vi "Create Space Image.vi"() -> ()   [LabVIEW 2020, in "Reversi.lvlib" / "Reversi.lvclass"]
uses:
  Reversi.lvclass
  Reversi.lvclass/Reversi.ctl
panel:
  out "White Space":picture
  out "Black Space":picture
  out "Blank Space":picture
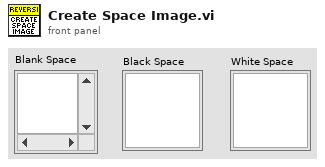
[diagram p1: front panel]
types:
  T1 = cluster{"left":i16, "top":i16, "right":i16, "bottom":i16}
  T2 = typedef "imagedata.ctl" = cluster{"image type":i32, "image depth":i32, "image":u8[], "mask":u8[], "colors":u32[], "Rectangle":cluster{"left":i16, "top":i16, "right":i16, "bottom":i16}}
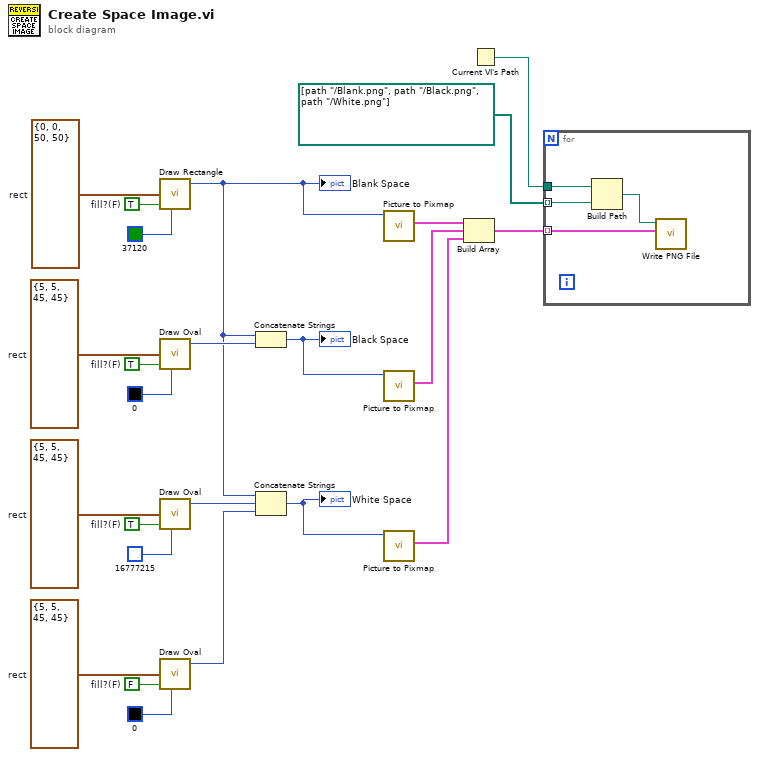
[diagram p0: block diagram]
diagram:
  w2 = FALSE  # fill?(F)
  w4 = T1 {"left"=5, "top"=5, "right"=45, "bottom"=45}  # rect
  w17 = TRUE  # fill?(F)
  w15 = T1 {"left"=5, "top"=5, "right"=45, "bottom"=45}  # rect
  w19 = TRUE  # fill?(F)
  w21 = T1 {"left"=5, "top"=5, "right"=45, "bottom"=45}  # rect
  w22 = TRUE  # fill?(F)
  w24 = T1 {"left"=0, "top"=0, "right"=50, "bottom"=50}  # rect
  n1 = call <vilib>:"Draw Rectangle.vi"("rect"=w24, "fill?(F)"=w22, "color(black)"=u32 37120) -> ("new picture"=w13:picture)  [unwired: 6 in]
  "Blank Space" <- w13
  n2 = call <vilib>:"Draw Oval.vi"("rect"=w21, "fill?(F)"=w19, "color(black)"=u32 0) -> ("new picture"=w18:picture)  [unwired: 6 in]
  n3 = call <vilib>:"Draw Oval.vi"("rect"=w15, "fill?(F)"=w17, "color(black)"=u32 16777215) -> ("new picture"=w14:picture)  [unwired: 6 in]
  n4 = call <vilib>:"Draw Oval.vi"("rect"=w4, "fill?(F)"=w2, "color(black)"=u32 0) -> ("new picture"=w1:picture)  [unwired: 6 in]
  n5 = Concatenate Strings(w13, w18) -> (w11:picture)
  "Black Space" <- w11
  n6 = Concatenate Strings(w13, w14, w1) -> (w10:picture)
  "White Space" <- w10
  n7 = call <vilib>:"Picture to Pixmap.vi"("picture"=w13) -> ("image data"=w12:T2)  [unwired: 9 in, 1 out]
  n8 = call <vilib>:"Picture to Pixmap.vi"("picture"=w11) -> ("image data"=w8:T2)  [unwired: 9 in, 1 out]
  n9 = call <vilib>:"Picture to Pixmap.vi"("picture"=w10) -> ("image data"=w7:T2)  [unwired: 9 in, 1 out]
  n10 = Build Array(w12, w8, w7) -> (w9:T2[])
  n11 = Current VI's Path() -> (path=w6:path)
  n12 = for {
    tunnel: w9 -> [w28] mode=indexing
    tunnel: w6 -> [w27]
    tunnel: path[] [path "../Blank.png", path "../Black.png", path "../White.png"] -> [w26] mode=indexing
    n13 = Build Path(base path=w27, name or relative path=w26) -> (appended path=w25:path)
    n14 = call <vilib>:"Write PNG File.vi"("image data"=w28, "path to PNG file"=w25) -> ()  [unwired: 8 in, 2 out]
  }
